vi "CANFD Set Schedule.vi"(5 "MsgTabNum":u8, 6 "pSendTimes":u16, 7 "pMsgNum":string, 9 "pCanMsgTab":T1, 10 "CANIndex":u8, 11 "DevHandle":i32) -> (1 "pCanMsgTab out":T1, 2 "function return":i32, 3 "pMsgNum out":string, 4 "pSendTimes out":u16)   [LabVIEW 2010, in "usb2canfd.lvlib"]
doc: "int WINAPI CANFD_SetSchedule(int DevHandle, unsigned char CANIndex, CANFD_MSG *pCanMsgTab,unsigned char *pMsgNum,unsigned short *pSendTimes,unsigned char MsgTabNum);"
uses:
  usb2canfd.lvlib
  USB2XXX/trunk/USB2XXX/USB2XXX/vs2019/Release/USB2XXX.dll
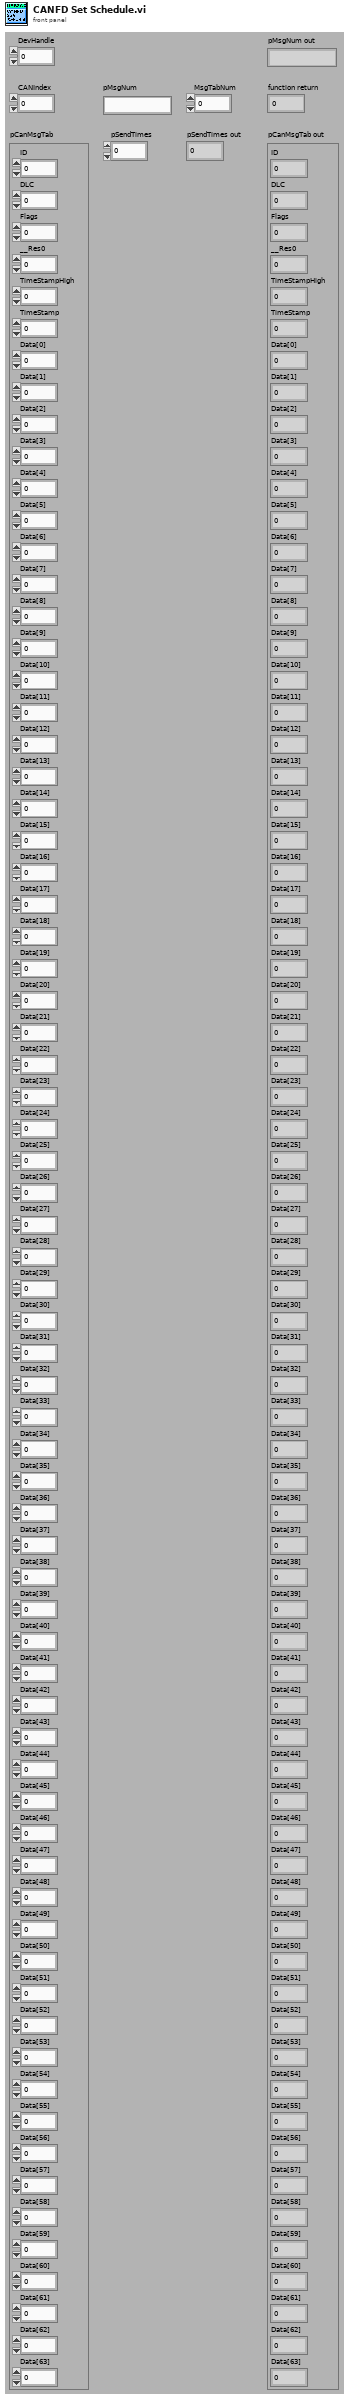
[diagram p1: front panel]
types:
  T1 = cluster{"ID":u32, "DLC":u8, "Flags":u8, "__Res0":u8, "TimeStampHigh":u8, "TimeStamp":u32, "Data[0]":u8, "Data[1]":u8, "Data[2]":u8, "Data[3]":u8, "Data[4]":u8, "Data[5]":u8, "Data[6]":u8, "Data[7]":u8, "Data[8]":u8, "Data[9]":u8, "Data[10]":u8, "Data[11]":u8, "Data[12]":u8, "Data[13]":u8, "Data[14]":u8, "Data[15]":u8, "Data[16]":u8, "Data[17]":u8, "Data[18]":u8, "Data[19]":u8, "Data[20]":u8, "Data[21]":u8, "Data[22]":u8, "Data[23]":u8, "Data[24]":u8, "Data[25]":u8, "Data[26]":u8, "Data[27]":u8, "Data[28]":u8, "Data[29]":u8, "Data[30]":u8, "Data[31]":u8, "Data[32]":u8, "Data[33]":u8, "Data[34]":u8, "Data[35]":u8, "Data[36]":u8, "Data[37]":u8, "Data[38]":u8, "Data[39]":u8, "Data[40]":u8, "Data[41]":u8, "Data[42]":u8, "Data[43]":u8, "Data[44]":u8, "Data[45]":u8, "Data[46]":u8, "Data[47]":u8, "Data[48]":u8, "Data[49]":u8, "Data[50]":u8, "Data[51]":u8, "Data[52]":u8, "Data[53]":u8, "Data[54]":u8, "Data[55]":u8, "Data[56]":u8, "Data[57]":u8, "Data[58]":u8, "Data[59]":u8, "Data[60]":u8, "Data[61]":u8, "Data[62]":u8, "Data[63]":u8}
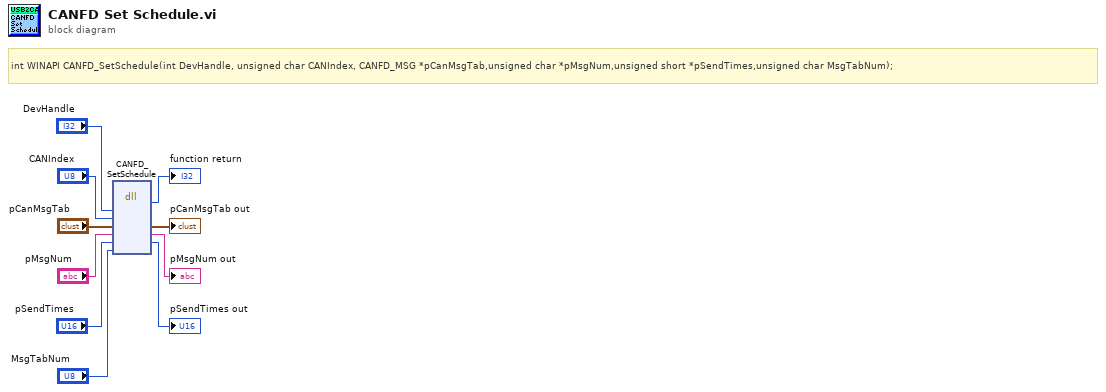
[diagram p0: block diagram]
diagram:
  # "int WINAPI CANFD_SetSchedule(int DevHandle, unsigned char CANIndex, CANFD_MSG *pCanMsgTab,unsigned char *pMsgNum,unsigned short *pSendTimes,unsigned char MsgTabNum);"
  n1 = dll-call lib="E:/Projects/USB2XXX/trunk/USB2XXX/USB2XXX/vs2019/Release/USB2XXX.*" fn="CANFD_SetSchedule"("DevHandle"="DevHandle", "CANIndex"="CANIndex", "pCanMsgTab"="pCanMsgTab", "pMsgNum"="pMsgNum", "pSendTimes"="pSendTimes", "MsgTabNum"="MsgTabNum") -> (→"function return":i32, "pCanMsgTab"=→"pCanMsgTab out":T1, "pMsgNum"=→"pMsgNum out":string, "pSendTimes"=→"pSendTimes out":u16)  [unwired: 6 in, 2 out]
